vi "Check Library Icon Data.vi"(6 "Expected Icon data":T1={"Text Visible?"=FALSE, "Text Opacity"=0, "Templ Visible?"=FALSE, "Templ Opacity"=0, "Relative Path from 1 to 2"=path "", "Image"=bytes[0], "All User Layers"=[], "Body Text"={"Line 1 text"="", "Line 2 text"="", "Line 3 text"="", "Line 4 text"="", "Line 1 color"=0, "Line 2 color"=0, "Line 3 color"=0, "Line 4 color"=0, "Body Text Spec"={"Font"="", "Alignment"=0, "Size"=3}, "Center text vertically"=FALSE, "Capitalize Text"=FALSE}} {"Body Text"."Body Text Spec"."Alignment" items=["left", "center", "right"]}, 8 "error in":errorcluster, 11 "Library Icon Data in":refnum<class "Library Icon Data.lvclass">) -> (0 "error out":errorcluster, 3 "Library Icon Data out":refnum<class "Library Icon Data.lvclass">)   [LabVIEW 2020, in "Library Icon Data.lvclass"]
doc: "Reads the icon data from the library and compares it to the expected data."
uses:
  Library Icon Data.lvclass
  Library Icon Data.lvclass/Library Icon Data.ctl
  e7d835d4-484a-418e-bbba-5da4f525552a.vi
  resource/plugins/lv_icon.lvlib
  vi.lib/LabVIEW Icon API/lv_icon/Controls/Alignment.ctl
  vi.lib/LabVIEW Icon API/lv_icon/Controls/Font.ctl
  vi.lib/LabVIEW Icon API/lv_icon/Controls/BodyText.ctl
  vi.lib/LabVIEW Icon API/lv_icon/Classes/Layer/Layer.lvclass
  vi.lib/LabVIEW Icon API/lv_icon/Controls/LabVIEW Icon Stored Information.ctl
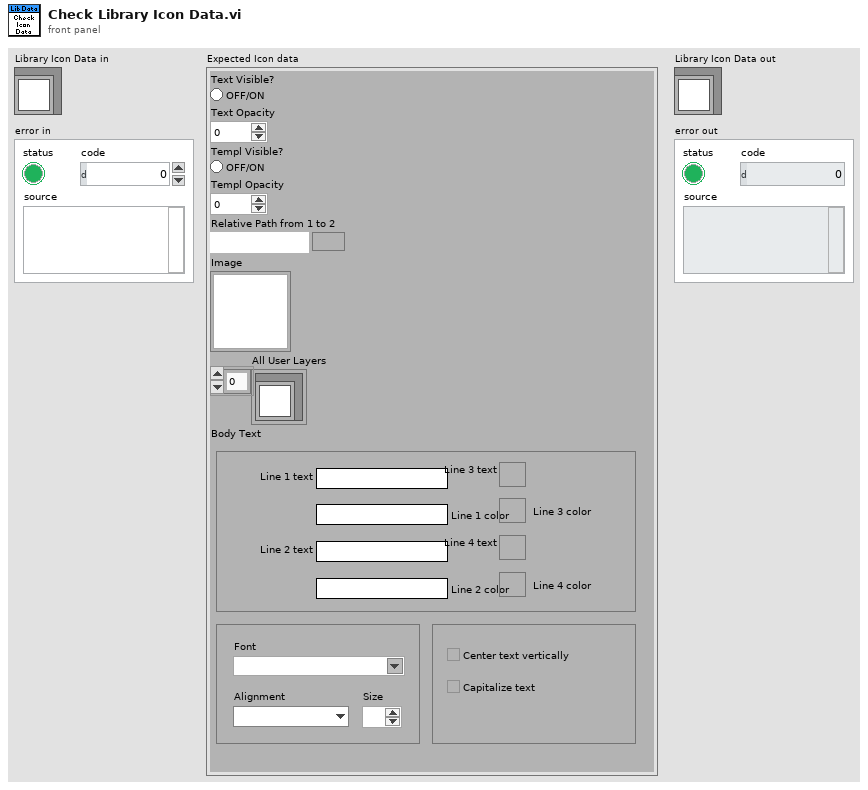
[diagram p1: front panel]
types:
  T1 = typedef "LabVIEW Icon Stored Information.ctl" = cluster{"Text Visible?":bool, "Text Opacity":u8, "Templ Visible?":bool, "Templ Opacity":u8, "Relative Path from 1 to 2":path, "Image":picture, "All User Layers":refnum<class "Layer.lvclass">[], "Body Text":T2}
  T2 = typedef "BodyText.ctl" = cluster{"Line 1 text":string, "Line 2 text":string, "Line 3 text":string, "Line 4 text":string, "Line 1 color":u32, "Line 2 color":u32, "Line 3 color":u32, "Line 4 color":u32, "Body Text Spec":cluster{"Font":T3, "Alignment":T4, "Size":u8}, "Center text vertically":bool, "Capitalize Text":bool}
  T3 = typedef "Font.ctl" = string
  T4 = typedef "Alignment.ctl" = u16
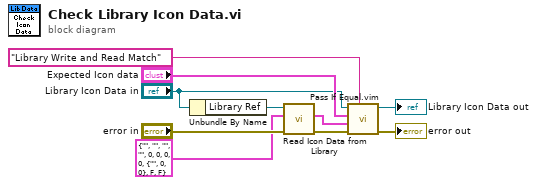
[diagram p0: block diagram]
diagram:
  n1 = Unbundle By Name("Library Icon Data in") -> ("Library Ref"=w5:refnum<vi>)
  n2 = call "Read Icon Data from Library.vi"("error in"="error in", "Default body text"=T2 {"Line 1 text"="", "Line 2 text"="", "Line 3 text"="", "Line 4 text"="", "Line 1 color"=0, "Line 2 color"=0, "Line 3 color"=0, "Line 4 color"=0, "Body Text Spec"={"Font"="", "Alignment"=0, "Size"=0}, "Center text vertically"=FALSE, "Capitalize Text"=FALSE}, "Library in"=w5) -> ("error out"=w9:errorcluster, "Data"=w2:T1)  [unwired: 6 in, 1 out]
  n3 = call "Pass If Equal.vim"("Description"="Library Write and Read Match", "error in (no error)"=w9, "Actual"=w2, "Expected"="Expected Icon data", "LUnit Test Case In"="Library Icon Data in") -> ("error out"=→"error out":errorcluster, "LUnit Test Case Out"=→"Library Icon Data out":refnum<class "Library Icon Data.lvclass">)  [unwired: 5 in]
